vi "Set Axis Properties.vi"(8 "error in (no error)":errorcluster, 10 "Axis Properties":T1, 11 "Scale Refnum":refnum<vi>) -> (0 "error out":errorcluster)   [LabVIEW 2020]
uses:
  Axis Properties.ctl
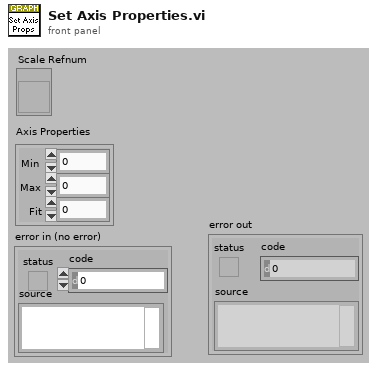
[diagram p1: front panel]
types:
  T1 = typedef "Axis Properties.ctl" = cluster{"Min":dbl, "Max":dbl, "Fit":u8}
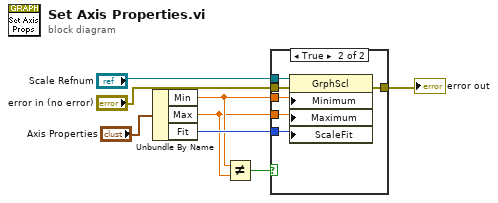
[diagram p0: block diagram]
diagram:
  n1 = Unbundle By Name("Axis Properties") -> ("Min"=w3:dbl, "Max"=w2:dbl, "Fit"=w4:u8)
  n2 = Not Equal?(x=w3, y=w2) -> (x != y?=w1:bool)
  n3 = case shown="True" w1 {
    tunnel: "Scale Refnum" -> [_ w15]
    tunnel: "error in (no error)" -> [w9 w14]
    tunnel: [w9 w13] -> w6
    tunnel: w4 -> [_ w12]
    tunnel: w3 -> [_ w11]
    tunnel: w2 -> [_ w10]
    frame False {
    }
    frame True {
      n4 = property class="GrphScl"(reference=w15, error in=w14, "Minimum"=w11, "Maximum"=w10, "ScaleFit"=w12) -> (error out=w13:errorcluster)  [unwired: 1 out]
    }
  }
  "error out" <- w6
